vi "Get Scanner.vi"(8 "error in (no error)":errorcluster, 11 "Translation Stages in":refnum<class "Translation Stages.lvclass">) -> (0 "error out":errorcluster, 2 "Default Scanner out":refnum<class "Scanner.lvclass">)   [LabVIEW 2012, in "Translation Stages.lvclass"]
doc: "(Dynamic) Returns the default Scanner object that scans over this Scannable. (Note that a Scannable may have multiple Scanners associated with it.) A Scanner is an analogue to an Iterator class in other languages."
uses:
  Translation Stages.lvclass
  Scanners/Scanner/Scanner.lvclass
  LabVIEW-programs/Instruments/Utility Classes/Scannable/Scannable.lvclass
  Scanners/Translation Stage/Translation Stage.lvclass
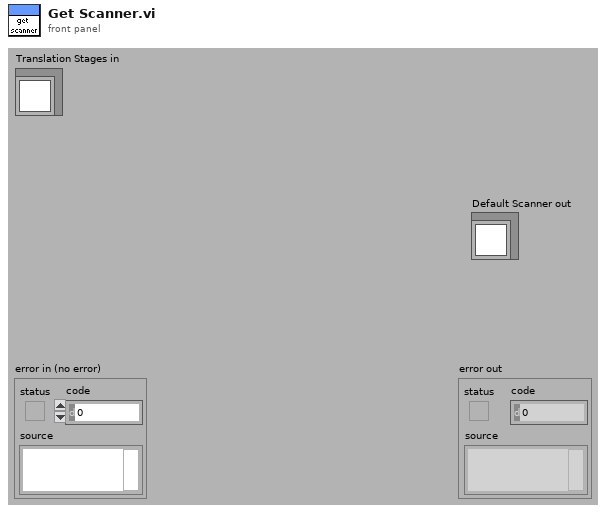
[diagram p1: front panel]
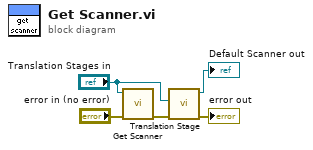
[diagram p0: block diagram]
diagram:
  n1 = call-parent "Get Scanner.vi"("error in (no error)"="error in (no error)", "Scannable in"="Translation Stages in") -> ("error out"=w2:errorcluster)  [unwired: 9 out]
  n2 = call "Translation Stage.vi"("error in (no error)"=w2, "Translation Stages.lvclass"="Translation Stages in") -> ("error out"=→"error out":errorcluster, "Translation Stage out"=→"Default Scanner out":refnum<class "Translation Stage.lvclass">)  [unwired: 8 out]
